vi "Open Transmission.vi"(8 "error in (no error)":errorcluster, 11 "TCPIP Communications in":refnum<class "TCPIP Communications.lvclass">) -> (0 "error out":errorcluster, 3 "TCPIP Communications out":refnum<class "TCPIP Communications.lvclass">)   [LabVIEW 2015, in "TCPIP Communications Framework.lvlib" / "TCPIP Communications.lvclass"]
uses:
  TCPIP Communications.lvclass
  TCPIP Communications.lvclass/TCPIP Communications.ctl
  <vilib>/ActorFramework/Actor/Actor.lvclass/Actor.ctl
  <vilib>/ActorFramework/Message Enqueuer/Message Enqueuer.lvclass/Message Enqueuer.ctl
  <vilib>/ActorFramework/Message Enqueuer/Init from Existing Queue.vi
  <vilib>/ActorFramework/Message Enqueuer/Enqueue.vi
  <vilib>/ActorFramework/Message Priority Queue/Priority Enqueue.vi
  <vilib>/ActorFramework/Message Enqueuer/Message Enqueuer.lvclass
  TCPIP Communications Messages/Open Transmission Msg/Open Transmission Msg.lvclass
  <vilib>/ActorFramework/Actor/Actor.lvclass
  Utilities/Status Messaging.llb/Status Messaging.lvlib
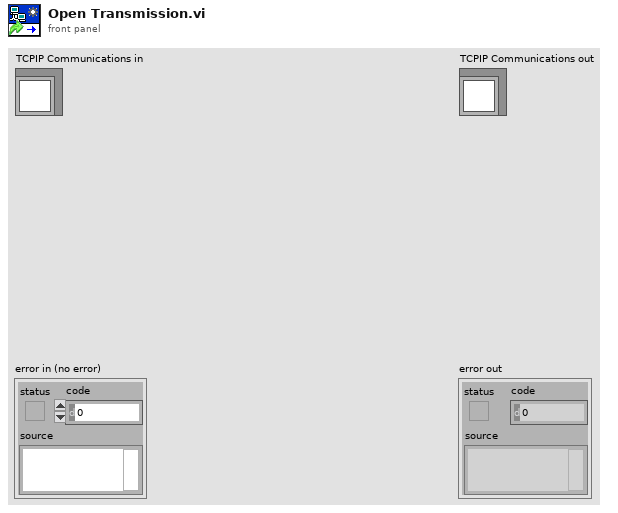
[diagram p1: front panel]
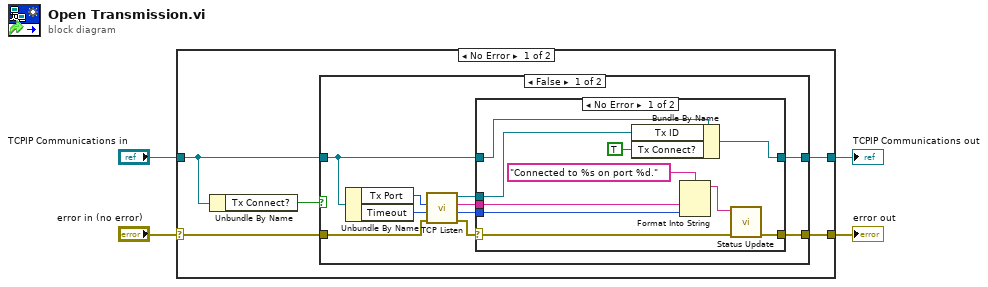
[diagram p0: block diagram]
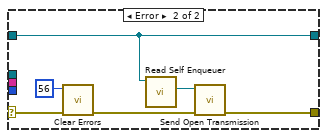
[diagram p2: hidden frame]
diagram:
  n1 = case shown="No Error" "error in (no error)" {
    selector: "error in (no error)" -> [w7 w39]
    tunnel: [w5 w39] -> w3
    tunnel: [w6 w38] -> w1
    tunnel: "TCPIP Communications in" -> [w9 w38]
    frame No Error {
      n2 = Unbundle By Name(w9) -> ("Tx Connect?"=w8:bool)
      n3 = case shown="False" w8 {
        tunnel: w9 -> [w16 w37]
        tunnel: w7 -> [w17 w36]
        tunnel: [w13 w37] -> w6
        tunnel: [w12 w36] -> w5
        frame False {
          n4 = Unbundle By Name(w16) -> ("Tx Port"=w19:u16, "Timeout"=w18:i32)
          n5 = call <vilib>:"TCP Listen.vi"("error in (no error)"=w17, "timeout ms (wait forever: -1)"=w18, "port"=w19) -> ("error out"=w15:errorcluster, "remote port"=w10:u16, "remote address"=w11:string, "connection ID"=w14:refnum<k5>)  [unwired: 4 in, 1 out]
          n6 = case shown="No Error" w15 {
            selector: w15 -> [w23 w35]
            tunnel: w16 -> [w29 w30]
            tunnel: w14 -> [w28 _]
            tunnel: [w27 w30] -> w13
            tunnel: [w22 w31] -> w12
            tunnel: w11 -> [w25 _]
            tunnel: w10 -> [w24 _]
            frame No Error {
              n7 = Bundle By Name(cluster=w29, "Tx ID"=w28, "Tx Connect?"=TRUE ("connected?")) -> (w27:refnum<class "TCPIP Communications.lvclass">)
              n8 = Format Into String(format string="Connected to %s on port %d." ("initial string"), w25, w24) -> (resulting string=w21:string)  [unwired: 2 in, 1 out]
              n9 = call "Status Update.vi"("error in (no error)"=w23, "Status Update"=w21) -> ("error out"=w22:errorcluster)  [unwired: 8 in, 1 out]
            }
            frame Error {
              n10 = call <vilib>:"Clear Errors.vi"("error in (no error)"=w35, "specific error code to clear (0: all)"=56) -> ("error out"=w32:errorcluster)  [unwired: 4 in, 1 out]
              n11 = call <vilib>:"Read Self Enqueuer.vi"("Actor"=w30) -> ("Self Enqueuer"=w33:refnum<class "Message Enqueuer.lvclass">)  [unwired: 10 in]
              n12 = call "Send Open Transmission.vi"("error in (no error)"=w32, "Message Enqueuer"=w33) -> ("error out"=w31:errorcluster)  [unwired: 8 in, 1 out]
            }
          }
        }
        frame True {
        }
      }
    }
    frame Error {
    }
  }
  "error out" <- w3
  "TCPIP Communications out" <- w1
